vi "GF_AddErrorArrays.vi"(1 "Error Array To Add In":errorcluster[](array[cluster]), 2 "Error Array In":errorcluster[](array[cluster])) -> (0 "Error Array Out":errorcluster[](array[cluster]))   [LabVIEW 2016]
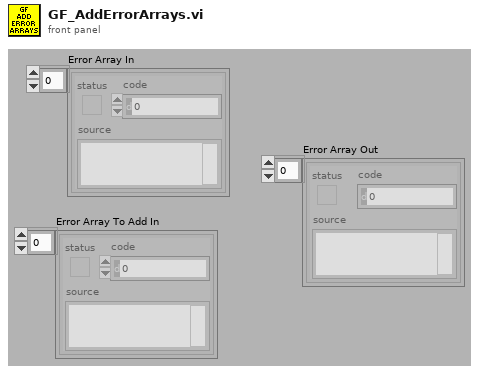
[diagram p1: front panel]
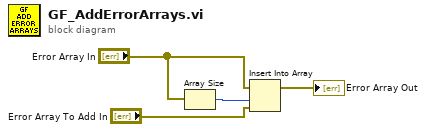
[diagram p0: block diagram]
diagram:
  n1 = Array Size(array="Error Array In") -> (size(s)=w2:i32)
  n2 = Insert Into Array(array="Error Array In", index=w2, new element="Error Array To Add In") -> (→"Error Array Out":errorcluster[])
